vi "Is Variant Type Boolean.vi"(8 "error in (no error)":errorcluster, 11 "variant":variant) -> (0 "error out":errorcluster, 2 "Type":T1=enum."Boolean", 3 "Is boolean?":bool)   [LabVIEW 2020, in "RxnRover.lvlib"]
doc: "Check if the variant contents are a boolean."
uses:
  RxnRover.lvlib
  Supported Parameter Variant Types.ctl
  <vilib>/Utility/Data Type/Type Definitions/Data Type.ctl
  <vilib>/Utility/Data Type/NI_Data Type.lvlib
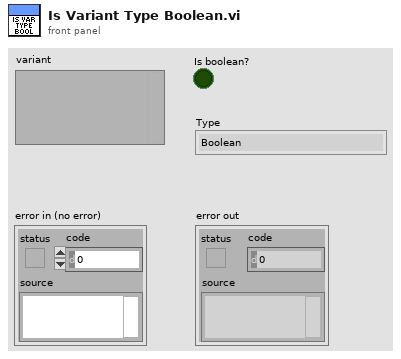
[diagram p1: front panel]
types:
  T1 = typedef "RxnRover.lvlib/Supported Parameter Variant Types.ctl" = enum16{"Unsupported", "Numeric", "Boolean", "String", "Path"}
  T2 = typedef "NI_Data Type.lvlib/Data Type.ctl" = enum8{"Invalid Type", "Void", "I8", "I16", "I32", "I64", "U8", "U16", "U32", "U64", "Single Float", "Double Float", "Extended Float", "Single Complex", "Double Complex", "Extended Complex", "Enum U8", "Enum U16", "Enum U32", "Enum U64", "Single Float With Unit", "Double Float With Unit", "Extended Float With Unit", "Single Complex with Unit", "Double Complex with Unit", "Extended Complex with Unit", "Boolean", "String", "Path", "Picture", "Tag", "Array", "Cluster", "Variant", "LV Variant", "Waveform", "Timestamp", "Digital Waveform", "Digital Data", "ExpressData", "Refnum", "External Data", "VI", "Poly VI", "LabVIEW Class Instance", "Fixed Point", "Set Collection", "Map Collection"}
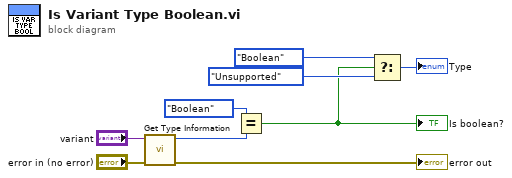
[diagram p0: block diagram]
diagram:
  n1 = call <vilib>:"Get Type Information.vi"("error in (no error)"="error in (no error)", "variant"="variant") -> ("error out"=→"error out":errorcluster, "type"=w5:T2)  [unwired: 5 in, 3 out]
  n2 = Equal?(x=Data_Type."Boolean" ("type"), y=w5) -> (x = y?=w1:bool)
  "Is boolean?" <- w1
  n3 = Select(t=Supported_Parameter_Variant_Types."Boolean" ("Supported Parameter Variant Types"), s=w1, f=Supported_Parameter_Variant_Types."Unsupported" ("Supported Parameter Variant Types")) -> (s? t:f=→"Type":T1)
